vi "SDG60RefClock.vi"(3 "Ref 10MHz Src (T: Int)":bool=TRUE, 4 "10MHz Out (T:Enable)":bool=TRUE) -> ()   [LabVIEW 2022 SP3]
doc: "Configures the output impedance and source impedance for the channel you specify."
uses:
  <vilib>/addons/zeromq/socket_type.ctl
  <vilib>/addons/zeromq/zmq_context.lvclass
  <vilib>/addons/zeromq/zmq_socket.lvclass
  <vilib>/addons/zeromq/zeromq.lvlib
panel:
  out "Python response":string
  # "If no valid external clock present,\noutputs will be switched off"
  # "Default state output state of\n10 MHz is off."
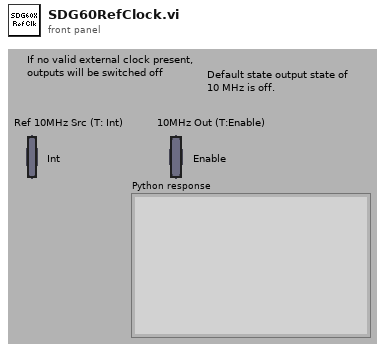
[diagram p1: front panel]
types:
  T1 = typedef "zeromq.lvlib/socket_type.ctl" = enum8{"ZMQ_PAIR", "ZMQ_PUB", "ZMQ_SUB", "ZMQ_REQ", "ZMQ_REP", "ZMQ_DEALER", "ZMQ_ROUTER", "ZMQ_PULL", "ZMQ_PUSH", "ZMQ_XPUB", "ZMQ_XSUB", "ZMQ_STREAM", "ZMQ_SERVER", "ZMQ_CLIENT", "ZMQ_RADIO", "ZMQ_DISH", "ZMQ_GATHER", "ZMQ_SCATTER", "ZMQ_DGRAM"}
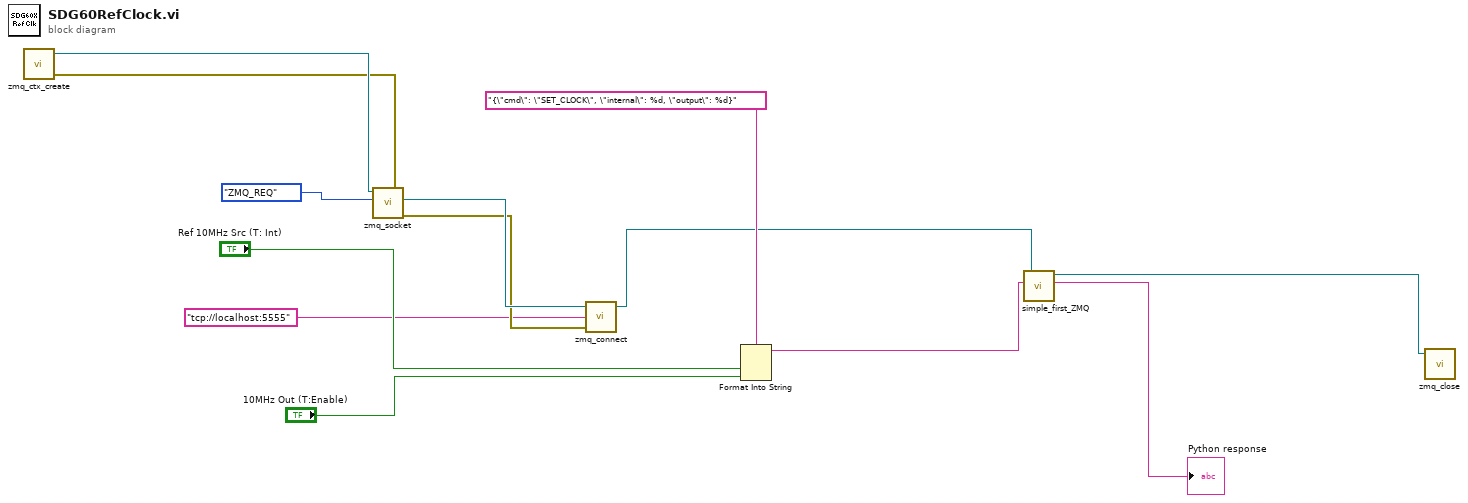
[diagram p0: block diagram]
diagram:
  n1 = call <vilib>:"zmq_ctx_create.vi"() -> ("error out"=w8:errorcluster, "context out"=w10:refnum<class "zmq_context.lvclass">)  [unwired: 4 in]
  n2 = call <vilib>:"zmq_socket.vi"("error in"=w8, "socket type"=socket_type."ZMQ_REQ", "context in"=w10) -> ("error out"=w7:errorcluster, "socket out"=w9:refnum<class "zmq_socket.lvclass">)  [unwired: 2 in, 1 out]
  n3 = call <vilib>:"zmq_connect.vi"("error in"=w7, "endpoint"="tcp://localhost:5555", "socket in"=w9) -> ("socket out"=w4:refnum<class "zmq_socket.lvclass">)  [unwired: 1 in, 1 out]
  n4 = Format Into String(format string="{\"cmd\": \"SET_CLOCK\", \"internal\": %d, \"output\": %d}", "Ref 10MHz Src (T: Int)", "10MHz Out (T:Enable)") -> (resulting string=w1:string)  [unwired: 2 in, 1 out]
  n5 = call "simple_first_ZMQ.vi"("Raw command"=w1, "ZMQ socket in"=w4) -> ("Python response"=→"Python response":string, "ZMQ socket out"=w3:refnum<class "zmq_socket.lvclass">)  [unwired: 4 in]
  n6 = call <vilib>:"zmq_close.vi"("socket"=w3) -> ()  [unwired: 4 in, 1 out]
